vi "NI-9381_SoftPanel.vi"(3 "NI-9381 in Slot:":string="1") -> ()   [LabVIEW 2016]
uses:
  GlobalControlVariables.vi
panel:
  out "ExitModule":bool=TRUE
  in  "DO 4":bool
  in  "DIO 4 Mode Select":string(combo)="Input"
  out "DI 4":bool
  in  "DO 3":bool
  in  "DIO 3 Mode Select":string(combo)="Input"
  out "DI 3":bool
  in  "DO 2":bool
  in  "DIO 2 Mode Select":string(combo)="Input"
  out "DI 2":bool
  out "AI 7":dbl
  out "AI 6":dbl
  out "AI 5":dbl
  out "AI 4":dbl
  out "AI 3":dbl
  out "AI 2":dbl
  out "AI 1":dbl
  out "AI 0":dbl
  in  "AO 7":dbl min=-10.0 max=10.0
  in  "AO 6":dbl min=-10.0 max=10.0
  in  "AO 5":dbl min=-10.0 max=10.0
  in  "AO 4":dbl min=-10.0 max=10.0
  in  "AO 3":dbl min=-10.0 max=10.0
  in  "AO 2":dbl min=-10.0 max=10.0
  in  "AO 1":dbl min=-10.0 max=10.0
  in  "AO 0":dbl min=-10.0 max=10.0
  in  "Submit DIO":bool
  in  "Submit AO":bool
  in  "DO 1":bool
  in  "DIO 1 Mode Select":string(combo)="Input"
  out "DI 1":bool
  in  "ExitButton":bool
  # "Analog Outputs"
  # "Analog Inputs"
  # "Digital IO"
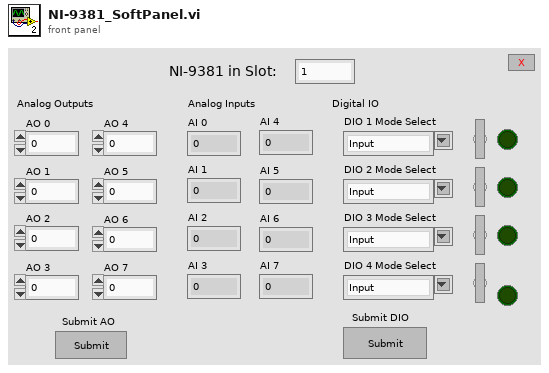
[diagram p1: front panel]
types:
  T1 = cluster{"TCP Analog Array[0]":dbl, "TCP Analog Array[1]":dbl, "TCP Analog Array[2]":dbl, "TCP Analog Array[3]":dbl, "TCP Analog Array[4]":dbl, "TCP Analog Array[5]":dbl, "TCP Analog Array[6]":dbl, "TCP Analog Array[7]":dbl}
  T2 = cluster{"Boolean array[0]":bool, "Boolean array[1]":bool, "Boolean array[2]":bool, "Boolean array[3]":bool}
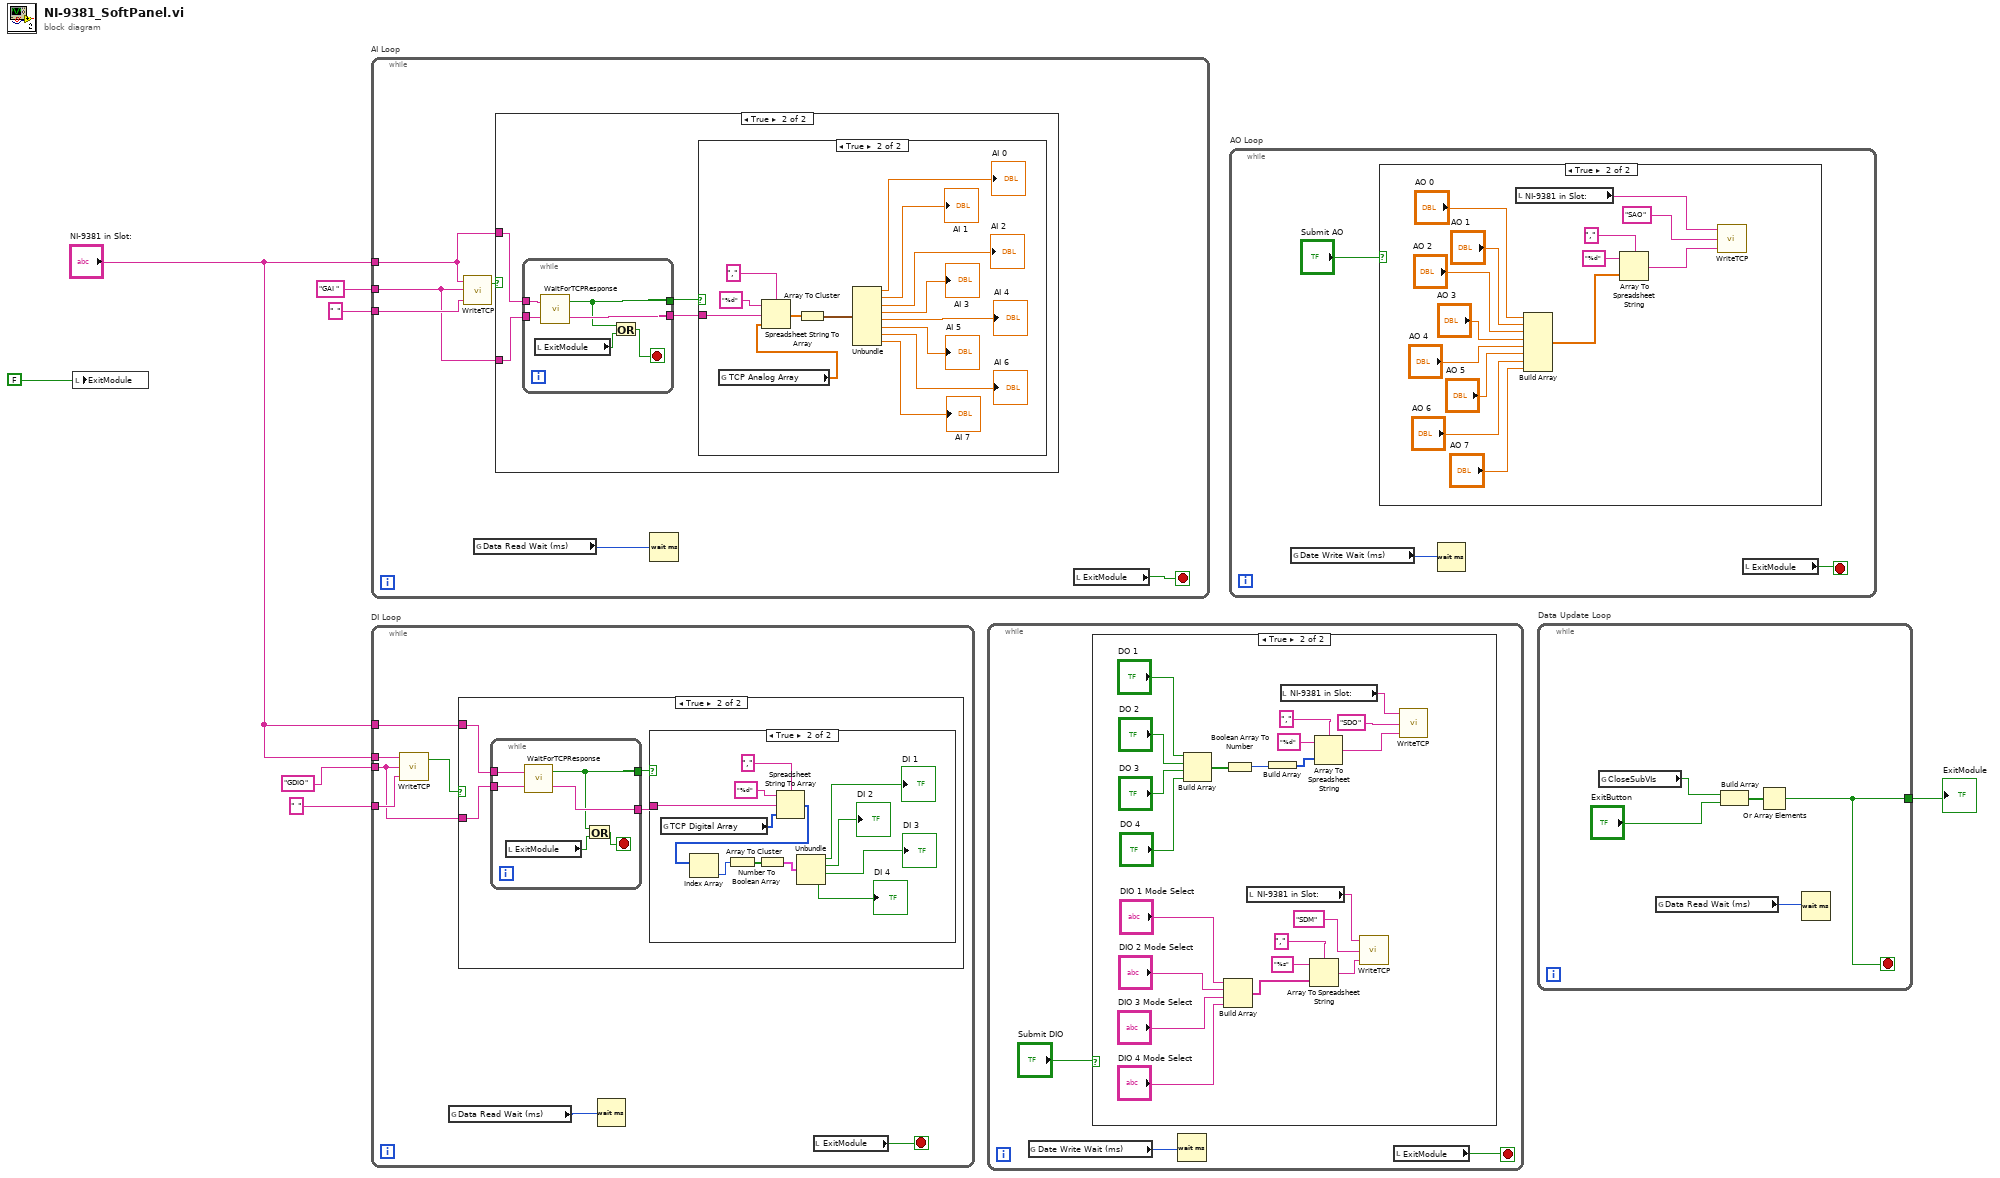
[diagram p0: block diagram]
diagram:
  n1 = local write "ExitModule"(FALSE) -> ()
  n2 = while "AI Loop" {
    tunnel: "NI-9381 in Slot:" -> [w11]
    tunnel: " " -> [w9]
    tunnel: "GAI " -> [w8]
    stop <- w13 stop-if-true
    n3 = call "WriteTCP.vi"("Data"=w9, "Action"=w8, "Module Slot"=w11) -> ("Sent"=w12:bool)  [unwired: 1 out]
    n4 = global read "GlobalControlVariables.vi" "Data Read Wait (ms)"() -> (w10:u32)
    n5 = case shown="True" w12 {
      tunnel: w11 -> [_ w16]
      tunnel: w8 -> [_ w15]
      frame False {
      }
      frame True {
        n6 = while {
          tunnel: [w18] -> w17
          tunnel: w16 -> [w23]
          tunnel: w15 -> [w22]
          tunnel: [w21] -> w14
          stop <- w19 stop-if-true
          n7 = local read "ExitModule"() -> (w20:bool)
          n8 = call "WaitForTCPResponse.vi"("Action"=w22, "Module Slot"=w23) -> ("Received Data"=w21:string, "Ready"=w18:bool)
          n9 = Or(x=w18, y=w20) -> (x .or. y?=w19:bool)
        }
        n10 = case shown="True" w17 {
          tunnel: w14 -> [_ w37]
          frame False {
          }
          frame True {
            n11 = global read "GlobalControlVariables.vi" "TCP Analog Array"() -> (w24:dbl[])
            n12 = Spreadsheet String To Array(delimiter (Tab)=",", format string="%d", spreadsheet string=w37, array type (2D Dbl)=w24) -> (array=w34:dbl[])
            n13 = Array To Cluster(array=w34) -> (cluster=w33:T1)
            n14 = Unbundle(w33) -> ("TCP Analog Array[0]"=→"AI 0":dbl, "TCP Analog Array[1]"=→"AI 1":dbl, "TCP Analog Array[2]"=→"AI 2":dbl, "TCP Analog Array[3]"=→"AI 3":dbl, "TCP Analog Array[4]"=→"AI 4":dbl, "TCP Analog Array[5]"=→"AI 5":dbl, "TCP Analog Array[6]"=→"AI 6":dbl, "TCP Analog Array[7]"=→"AI 7":dbl)
          }
        }
      }
    }
    n15 = Wait (ms)(milliseconds to wait=w10) -> ()  [unwired: 1 out]
    n16 = local read "ExitModule"() -> (w13:bool)
  }
  n17 = while "DI Loop" {
    tunnel: "NI-9381 in Slot:" -> [w43]
    tunnel: "NI-9381 in Slot:" -> [w41]
    tunnel: "GDIO" -> [w38]
    tunnel: " " -> [w39]
    stop <- w44 stop-if-true
    n18 = call "WriteTCP.vi"("Data"=w39, "Action"=w38, "Module Slot"=w43) -> ("Sent"=w42:bool)  [unwired: 1 out]
    n19 = global read "GlobalControlVariables.vi" "Data Read Wait (ms)"() -> (w40:u32)
    n20 = case shown="True" w42 {
      tunnel: w41 -> [_ w48]
      tunnel: w38 -> [_ w45]
      frame False {
      }
      frame True {
        n21 = while {
          tunnel: w48 -> [w54]
          tunnel: [w49] -> w47
          tunnel: [w53] -> w46
          tunnel: w45 -> [w52]
          stop <- w51 stop-if-true
          n22 = local read "ExitModule"() -> (w50:bool)
          n23 = call "WaitForTCPResponse.vi"("Action"=w52, "Module Slot"=w54) -> ("Received Data"=w53:string, "Ready"=w49:bool)
          n24 = Or(x=w49, y=w50) -> (x .or. y?=w51:bool)
        }
        n25 = case shown="True" w47 {
          tunnel: w46 -> [_ w63]
          frame False {
          }
          frame True {
            n26 = global read "GlobalControlVariables.vi" "TCP Digital Array"() -> (w64:u32[])
            n27 = Spreadsheet String To Array(delimiter (Tab)=",", format string="%d", spreadsheet string=w63, array type (2D Dbl)=w64) -> (array=w62:u32[])
            n28 = Index Array(array=w62) -> (element=w61:u32)  [unwired: 1 in]
            n29 = Number To Boolean Array(number=w61) -> (Boolean array=w60:bool[])
            n30 = Array To Cluster(array=w60) -> (cluster=w59:T2)
            n31 = Unbundle(w59) -> ("Boolean array[0]"=→"DI 1":bool, "Boolean array[1]"=→"DI 2":bool, "Boolean array[2]"=→"DI 3":bool, "Boolean array[3]"=→"DI 4":bool)
          }
        }
      }
    }
    n32 = Wait (ms)(milliseconds to wait=w40) -> ()  [unwired: 1 out]
    n33 = local read "ExitModule"() -> (w44:bool)
  }
  n34 = while {
    stop <- w68 stop-if-true
    n35 = global read "GlobalControlVariables.vi" "Date Write Wait (ms)"() -> (w67:u32)
    n36 = case shown="True" "Submit DIO" {
      frame False {
      }
      frame True {
        n37 = Build Array("DO 1", "DO 2", "DO 3", "DO 4") -> (w83:bool[])
        n38 = Build Array("DIO 1 Mode Select", "DIO 2 Mode Select", "DIO 3 Mode Select", "DIO 4 Mode Select") -> (w73:string[])
        n39 = Boolean Array To Number(Boolean array=w83) -> (number=w76:u32)
        n40 = local read "NI-9381 in Slot:"() -> (w70:string)
        n41 = Build Array(w76) -> (w75:u32[])
        n42 = local read "NI-9381 in Slot:"() -> (w71:string)
        n43 = Array To Spreadsheet String(delimiter (Tab)=",", array=w73, 3:"%s") -> (spreadsheet string=w77:string)
        n44 = Array To Spreadsheet String(delimiter (Tab)=",", array=w75, 3:"%d") -> (spreadsheet string=w80:string)
        n45 = call "WriteTCP.vi"("Data"=w77, "Action"="SDM", "Module Slot"=w70) -> ()  [unwired: 2 out]
        n46 = call "WriteTCP.vi"("Data"=w80, "Action"="SDO", "Module Slot"=w71) -> ()  [unwired: 2 out]
      }
    }
    n47 = Wait (ms)(milliseconds to wait=w67) -> ()  [unwired: 1 out]
    n48 = local read "ExitModule"() -> (w68:bool)
  }
  n49 = while "AO Loop" {
    stop <- w92 stop-if-true
    n50 = global read "GlobalControlVariables.vi" "Date Write Wait (ms)"() -> (w93:u32)
    n51 = case shown="True" "Submit AO" {
      frame False {
      }
      frame True {
        n52 = local read "NI-9381 in Slot:"() -> (w97:string)
        n53 = Build Array("AO 0", "AO 1", "AO 2", "AO 3", "AO 4", "AO 5", "AO 6", "AO 7") -> (w98:dbl[])
        n54 = Array To Spreadsheet String(delimiter (Tab)=",", array=w98, 3:"%d") -> (spreadsheet string=w96:string)
        n55 = call "WriteTCP.vi"("Data"=w96, "Action"="SAO", "Module Slot"=w97) -> ()  [unwired: 2 out]
      }
    }
    n56 = Wait (ms)(milliseconds to wait=w93) -> ()  [unwired: 1 out]
    n57 = local read "ExitModule"() -> (w92:bool)
  }
  n58 = while "Data Update Loop" {
    tunnel: [w109] -> w1
    stop <- w109 stop-if-true
    n59 = global read "GlobalControlVariables.vi" "CloseSubVIs"() -> (w110:bool)
    n60 = global read "GlobalControlVariables.vi" "Data Read Wait (ms)"() -> (w113:u32)
    n61 = Build Array(w110, "ExitButton") -> (w112:bool[])
    n62 = Or Array Elements(Boolean array=w112) -> (logical OR=w109:bool)
    n63 = Wait (ms)(milliseconds to wait=w113) -> ()  [unwired: 1 out]
  }
  "ExitModule" <- w1
